vi "Rabi.vi"() -> ()   [LabVIEW 2017]
uses:
  Expose/Labview/Parameters/ExposeParameterBindingType.ctl
  Experiment/ExpGet.vi
  Expose/Labview/Core/ExposeInvokeMethod.vi
  <userlib>/_OpenG.lib/lvdata/lvdata.llb/Get Default Data from Variant__ogtk.vi
panel:
  in  "btnAbort":bool
  in  "btnRunRabi":bool
  in  "Results":T1
  in  "ScanProperties":T2={"PiStartT"=0.0, "PiEndT"=1.0, "N"=100.0, "RepCount"=100, "DoAvg"=TRUE} caption="Scan" {"RepCount" min=1 max=10000000; "N" min=0.0 step=0.1; "PiEndT" min=0.0 step=0.1; "PiStartT" min=0.0 step=0.1}
  in  "RFProperties":cluster{"Amplitude":dbl, "Frequency":dbl}={"Amplitude"=-30.0, "Frequency"=0.0} caption="RF" {"Frequency" min=0.0; "Amplitude" max=12.0}
  in  "SystemConfig":T3={"MTriggerChannel"=1, "FGTriggerChannel"=2, "UseFG"=TRUE, "UseLaser"=TRUE, "UseRF"=TRUE, "LaserChannel"=3, "RFChannel"=4, "UseAnalogInputA0"=FALSE} caption="System" {"RFChannel" min=1 max=32 step=1; "LaserChannel" min=1 max=32 step=1; "FGTriggerChannel" min=1 max=32 step=1; "MTriggerChannel" min=1 max=32 step=1}
  in  "GateDisplay":cluster{"amp":dbl[][], "dt":dbl}
  in  "ReaderProperties":cluster{"BinsPerFreq":u32, "MaxFreq":dbl}={"BinsPerFreq"=1, "MaxFreq"=100000000.0} caption="Reader" {"MaxFreq" min=0.0 step=0.1; "BinsPerFreq" min=1 max=10000}
  in  "TimeProperties":T4={"InitT"=3.0, "WaitForPI"=0.5, "ReadT"=0.25, "WaitAfterPI"=0.5, "WaitForReferenceT"=2.0, "ReadLaserT"=5.0, "WaitAfterMeasurement"=2.0, "LaserDelay"=5.0} caption="Rabi Times" {"LaserDelay" min=0.0 step=0.1; "WaitAfterMeasurement" min=0.0 step=0.1; "ReadLaserT" min=0.0 step=0.1; "WaitForReferenceT" min=0.0 step=0.1; "WaitAfterPI" min=0.0 step=0.1; "ReadT" min=0.0 step=0.1; "WaitForPI" min=0.0 step=0.1; "InitT" min=0.0 step=0.1}
  out "LastBinIndex":dbl caption="#" format="%_7g"
  out "PendingRepetitionCount":dbl caption="Rem." format="%_7g"
  out "BinIndexIndicator":dbl(slide) max=201.0 step=1.0 scale=0.0..1.0
  out "PendingRepIndcator":dbl(slide) max=3.0 step=1.0 scale=0.0..1.0
  out "GraphYPosition":dbl caption="Y" format="%_7g"
  out "GraphXPosition":dbl caption="X" format="%_7g"
  out "IsWorking":bool=TRUE
  out "ExpID":string="Exp967f258c607eed45caf40f4c3101458dC" caption="Exp. ID (Debug)"
  out "ResultsGraph":T5(graph)
  out "MeanStreamVal":dbl caption="M. Ampl." format="%_7g"
  in  "ReadTickTime":dbl
  out "Stream":dbl[](graph) caption="Counts"
  out "TriggersGraph":digitalwaveform(graph)
  # "[¶ scan goes here]"
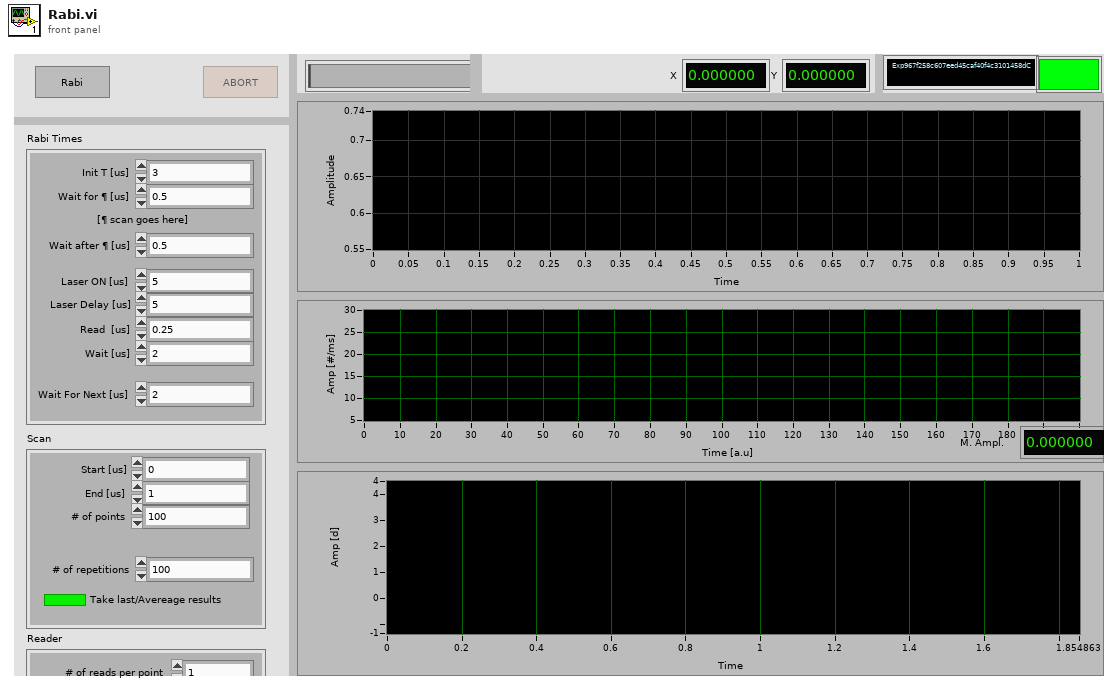
[diagram p1: front panel]
types:
  T1 = cluster{"StepSize":dbl, "Amps":dbl[], "StartOffset":dbl, "Reference":dbl[]}
  T2 = cluster{"PiStartT":dbl, "PiEndT":dbl, "N":dbl, "RepCount":u32, "DoAvg":bool}
  T3 = cluster{"MTriggerChannel":u32, "FGTriggerChannel":u32, "UseFG":bool, "UseLaser":bool, "UseRF":bool, "LaserChannel":u32, "RFChannel":u32, "UseAnalogInputA0":bool}
  T4 = cluster{"InitT":dbl, "WaitForPI":dbl, "ReadT":dbl, "WaitAfterPI":dbl, "WaitForReferenceT":dbl, "ReadLaserT":dbl, "WaitAfterMeasurement":dbl, "LaserDelay":dbl}
  T5 = cluster{dbl, "Frequencies":dbl, "Frequencies":dbl}[]
  T6 = enum8{"Enabled", "Disabled", "Disabled and Grayed Out"}
  T7 = typedef "ExposeParameterBindingType.ctl" = enum16{"ToRemote", "FromRemote", "Bidrectional"}
  T8 = cluster{dbl, "Frequencies":dbl, "Frequencies":dbl}
  T9 = typedef "LVPoint32TypeDef.ctl" = cluster{"Horizontal":i32, "Vertical":i32}
  T10 = typedef "LVRectTypeDef.ctl" = cluster{"Left":i16, "Top":i16, "Right":i16, "Bottom":i16}
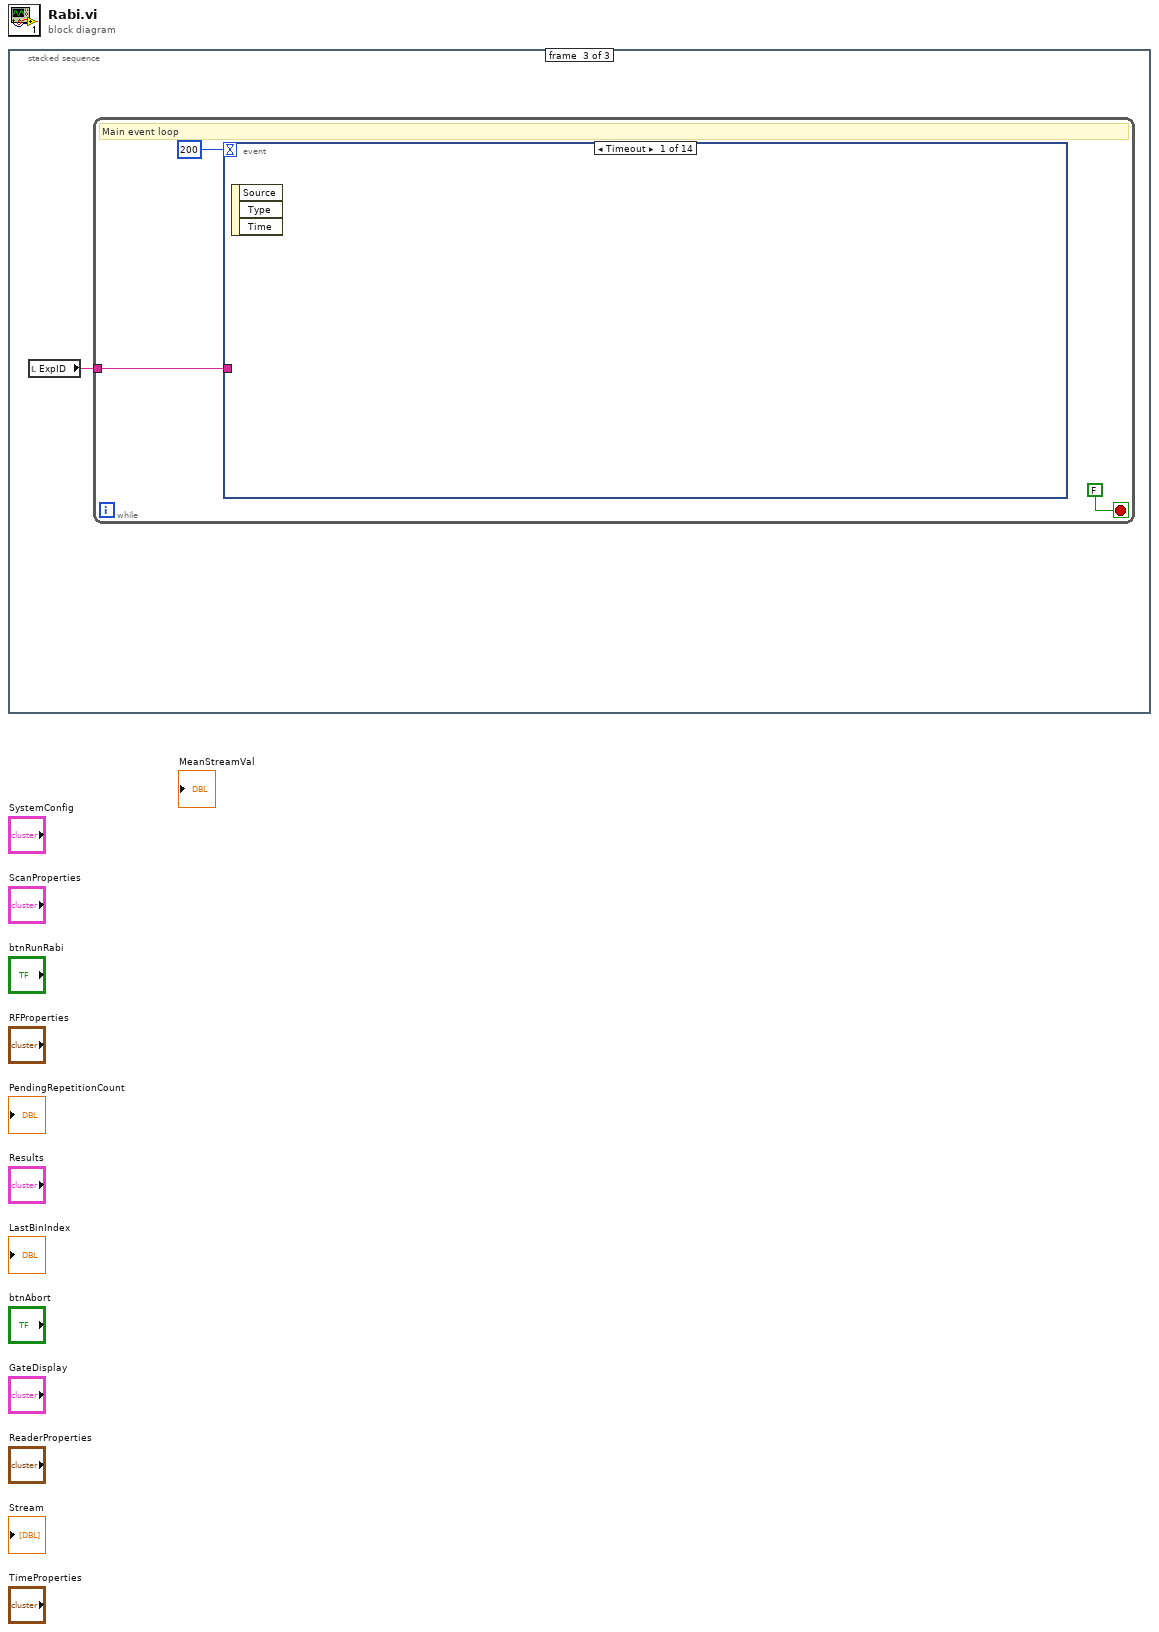
[diagram p0: block diagram]
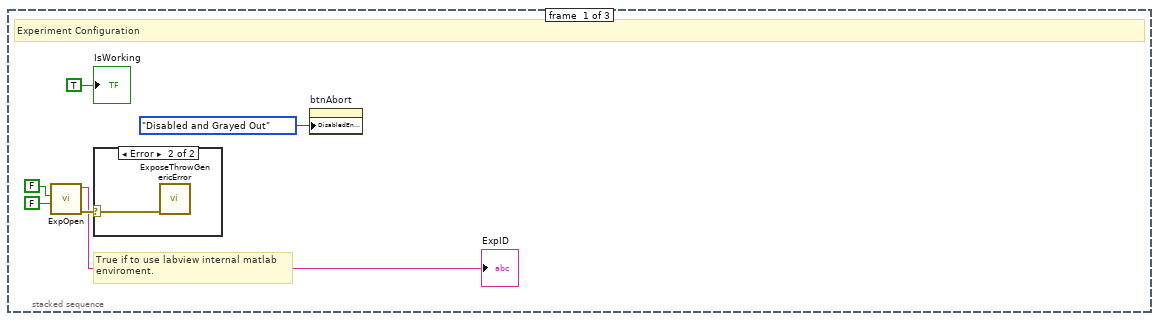
[diagram p2: hidden frame]
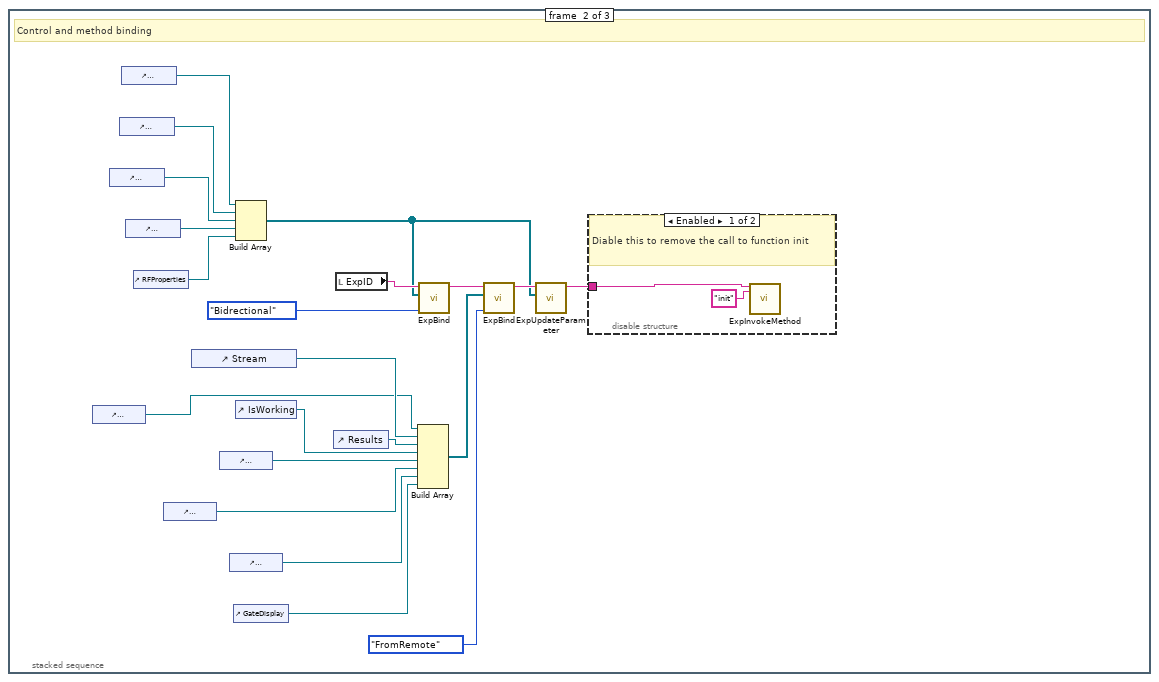
[diagram p4: hidden frame]
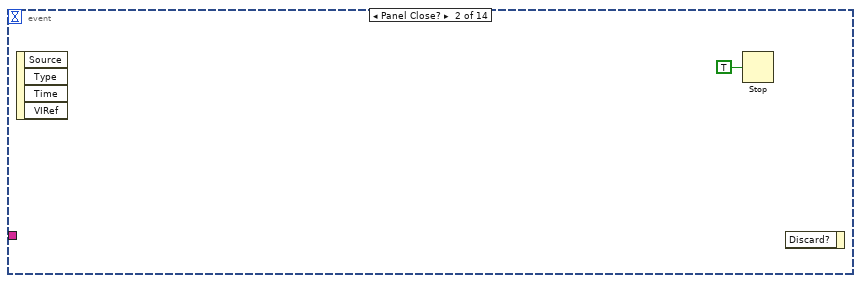
[diagram p6: hidden frame]
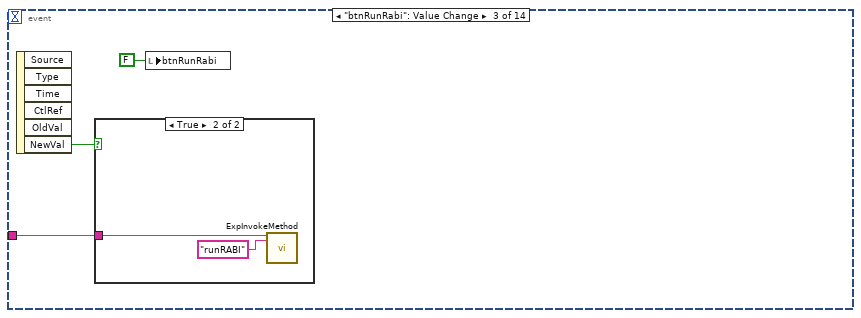
[diagram p7: hidden frame]
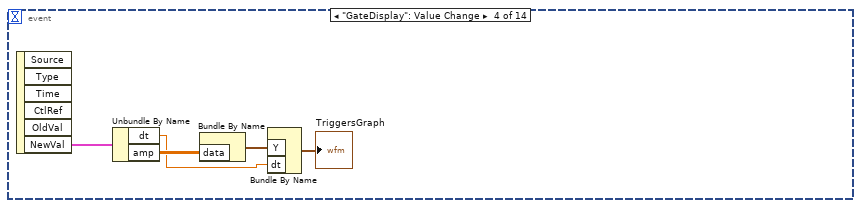
[diagram p9: hidden frame]
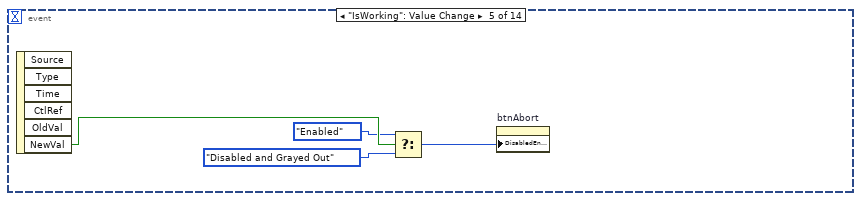
[diagram p10: hidden frame]
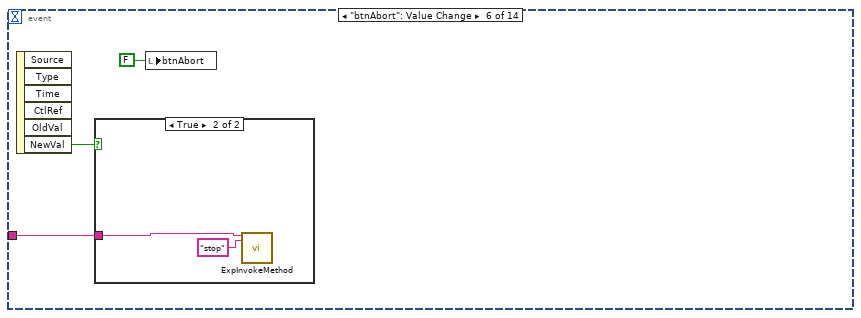
[diagram p11: hidden frame]
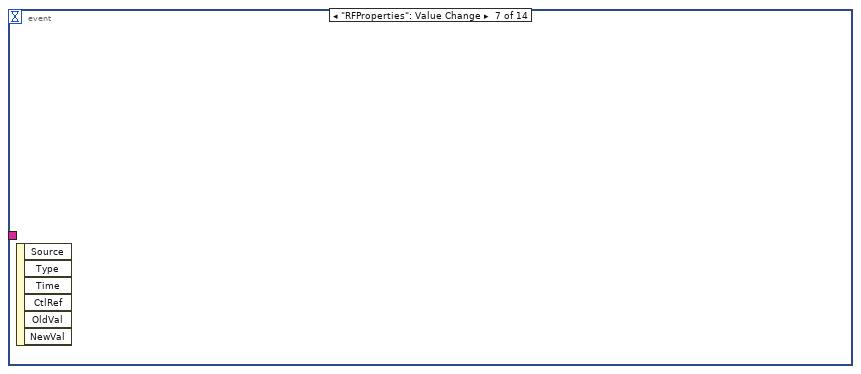
[diagram p13: hidden frame]
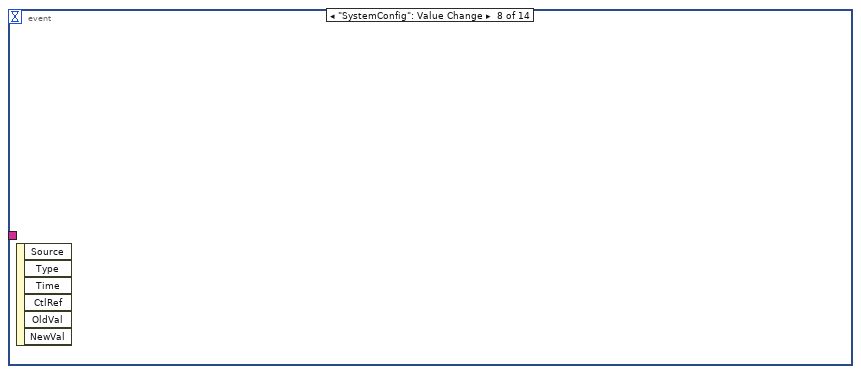
[diagram p14: hidden frame]
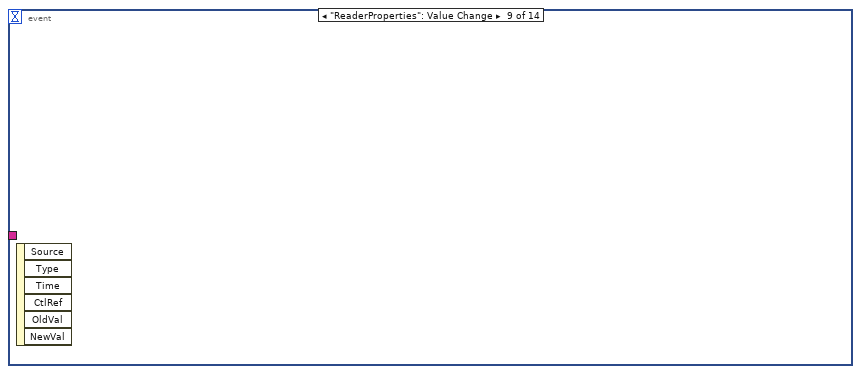
[diagram p15: hidden frame]
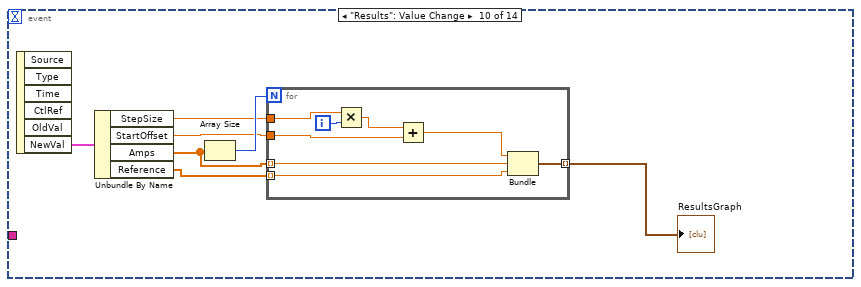
[diagram p16: hidden frame]
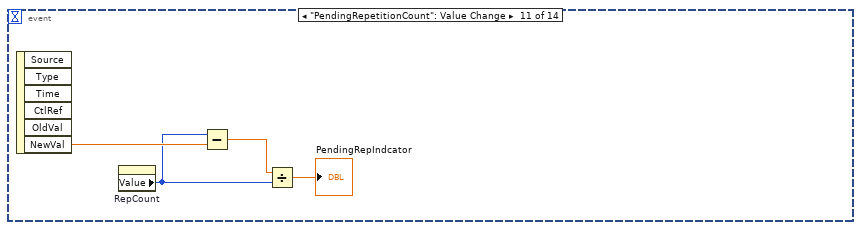
[diagram p17: hidden frame]
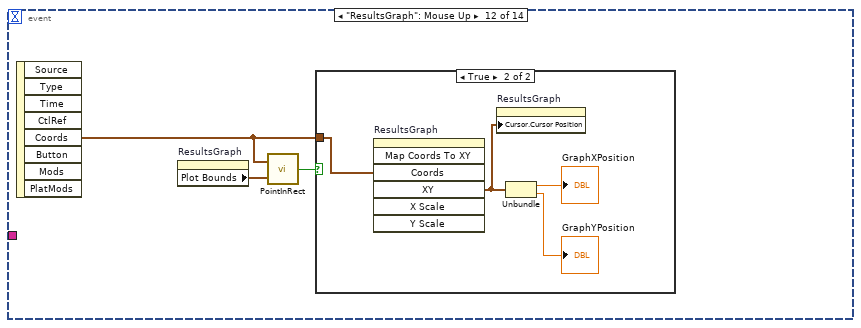
[diagram p18: hidden frame]
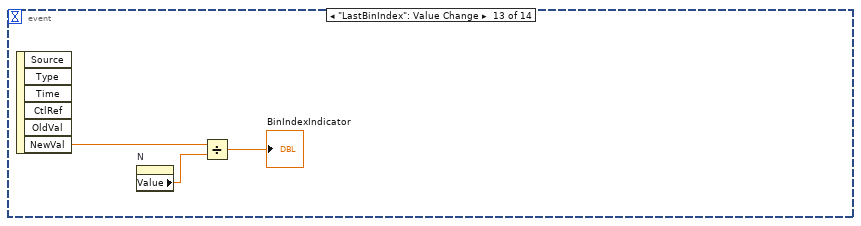
[diagram p20: hidden frame]
diagram:
  n1 = stacked-sequence {
    frame #0 {
      # "True if to use labview internal matlab\nenviroment."
      # "Experiment Configuration"
      n2 = call "ExpOpen.vi"("Do Expose Logging"=FALSE, "Requires Matlab Enviroment"=FALSE) -> ("error out"=w4:errorcluster, "ExpID"=→"ExpID":string)  [unwired: 7 in, 1 out]
      n3 = case shown="Error" w4 {
        selector: w4 -> [_ w7]
        frame No Error {
        }
        frame Error {
          n4 = call "ExposeThrowGenericError.vi"("error in (no error)"=w7) -> ()  [unwired: 10 in, 1 out]
        }
      }
      n5 = property on="btnAbort" class="Bool (strict)"("DisabledEnum"=T6."Disabled and Grayed Out" ("Disabled")) -> ()  [unwired: 2 in, 2 out]
      "IsWorking" <- TRUE ("IsWorking")
    }
    frame #1 {
      # "Control and method binding"
      n6 = control-ref of="MeanStreamVal"() -> (w8:refnum<vi>)
      n7 = control-ref of="ReaderProperties"() -> (w19:refnum<vi>)
      n8 = control-ref of="TimeProperties"() -> (w18:refnum<vi>)
      n9 = control-ref of="ScanProperties"() -> (w10:refnum<vi>)
      n10 = control-ref of="SystemConfig"() -> (w12:refnum<vi>)
      n11 = control-ref of="RFProperties"() -> (w11:refnum<vi>)
      n12 = control-ref of="PendingRepetitionCount"() -> (w15:refnum<vi>)
      n13 = control-ref of="Stream"() -> (w25:refnum<vi>)
      n14 = control-ref of="ReadTickTime"() -> (w17:refnum<vi>)
      n15 = control-ref of="LastBinIndex"() -> (w14:refnum<vi>)
      n16 = control-ref of="GateDisplay"() -> (w13:refnum<vi>)
      n17 = Build Array(w10, w18, w19, w12, w11) -> (w16:refnum<vi>[])
      n18 = control-ref of="IsWorking"() -> (w23:refnum<vi>)
      n19 = control-ref of="Results"() -> (w9:refnum<vi>)
      n20 = local read "ExpID"() -> (w28:string)
      n21 = Build Array(w8, w25, w9, w23, w17, w15, w14, w13) -> (w24:refnum<vi>[])
      n22 = call "ExpBind.vi"("Binding Type"=ExposeParameterBindingType."Bidrectional", "Value"=w16, "ExpID"=w28) -> ("ExpID out"=w21:string)  [unwired: 7 in, 1 out]
      n23 = call "ExpBind.vi"("Binding Type"=ExposeParameterBindingType."FromRemote", "Value"=w24, "ExpID"=w21) -> ("ExpID out"=w20:string)  [unwired: 7 in, 1 out]
      n24 = call "ExpUpdateParameter.vi"("Variant"=w16, "ExpID"=w20) -> ("ExpID out"=w22:string)  [unwired: 8 in, 1 out]
      n25 = disable-structure shown="Enabled" {
        disable-tunnel: w22 -> [w30 _]
        frame Enabled {
          # "Diable this to remove the call to function init"
          n26 = call "ExpInvokeMethod.vi"("ExpID"=w30, "Method Name"="init") -> ()  [unwired: 15 in, 3 out]
        }
        frame Disabled {
        }
      }
    }
    frame #2 {
      n27 = local read "ExpID"() -> (w31:string)
      n28 = while {
        tunnel: w31 -> [w32]
        stop <- FALSE stop-if-true
        # "Main event loop"
        n29 = event shown="[0] Timeout" {
          selector: _ -> [_ _ _ _ _ _ _ _ _ _ _ _ _ _]
          dyn-events: _ -> [_ _ _ _ _ _ _ _ _ _ _ _ _ _]
          timeout: 200 -> [_ _ _ _ _ _ _ _ _ _ _ _ _ _]
          tunnel: w32 -> [_ _ w38 _ _ w51 _ _ _ _ _ _ _ _]
          event Timeout {
            n30 = event-data() -> ()  [unwired: 1 in, 3 out]
          }
          event Panel Close? {
            n31 = event-data() -> ()  [unwired: 1 in, 4 out]
            n32 = Stop(stop? (T)=TRUE) -> ()
            n33 = event-data() -> ()  [unwired: 2 in, 1 out]
          }
          event "btnRunRabi": Value Change {
            n34 = event-data() -> ("NewVal"=w37:bool)  [unwired: 1 in, 5 out]
            n35 = case shown="True" w37 {
              tunnel: w38 -> [_ w40]
              frame False {
              }
              frame True {
                n36 = call "ExpInvokeMethod.vi"("ExpID"=w40, "Method Name"="runRABI") -> ()  [unwired: 15 in, 3 out]
              }
            }
            n37 = local write "btnRunRabi"(FALSE ("btnRunOdmr")) -> ()
          }
          event "GateDisplay": Value Change {
            n38 = event-data() -> ("NewVal"=w45:cluster{"amp":dbl[][], "dt":dbl})  [unwired: 1 in, 5 out]
            n39 = Unbundle By Name(w45) -> ("dt"=w43:dbl, "amp"=w44:dbl[][])
            n40 = Bundle By Name("data"=w44) -> (w42:digitaldata)  [unwired: 1 in]
            n41 = Bundle By Name("Y"=w42, "dt"=w43) -> (→"TriggersGraph":digitalwaveform)  [unwired: 1 in]
          }
          event "IsWorking": Value Change {
            n42 = event-data() -> ("NewVal"=w49:bool)  [unwired: 1 in, 5 out]
            n43 = Select(t=T6."Enabled" ("Disabled"), s=w49, f=T6."Disabled and Grayed Out" ("Disabled")) -> (s? t:f=w46:T6)
            n44 = property on="btnAbort" class="Bool (strict)"("DisabledEnum"=w46) -> ()  [unwired: 2 in, 2 out]
          }
          event "btnAbort": Value Change {
            n45 = event-data() -> ("NewVal"=w52:bool)  [unwired: 1 in, 5 out]
            n46 = case shown="True" w52 {
              tunnel: w51 -> [_ w54]
              frame False {
              }
              frame True {
                n47 = call "ExpInvokeMethod.vi"("ExpID"=w54, "Method Name"="stop") -> ()  [unwired: 15 in, 3 out]
              }
            }
            n48 = local write "btnAbort"(FALSE ("btnAbort")) -> ()
          }
          event "RFProperties": Value Change {
            n49 = event-data() -> ()  [unwired: 1 in, 6 out]
          }
          event "SystemConfig": Value Change {
            n50 = event-data() -> ()  [unwired: 1 in, 6 out]
          }
          event "ReaderProperties": Value Change {
            n51 = event-data() -> ()  [unwired: 1 in, 6 out]
          }
          event "Results": Value Change {
            n52 = event-data() -> ("NewVal"=w61:T1)  [unwired: 1 in, 5 out]
            n53 = Unbundle By Name(w61) -> ("StepSize"=w58:dbl, "StartOffset"=w59:dbl, "Amps"=w57:dbl[], "Reference"=w56:dbl[])
            n54 = Array Size(array=w57) -> (size(s)=w60:i32)
            n55 = for {
              N: w60 -> [_]
              tunnel: w59 -> [w69]
              tunnel: w58 -> [w67]
              tunnel: w57 -> [w65] mode=indexing
              tunnel: w56 -> [w62] mode=indexing
              tunnel: [w64] -> w55 mode=indexing
              i -> [w68]
              n56 = Multiply(x=w67, y=w68) -> (x*y=w66:dbl)
              n57 = Add(x=w66, y=w69) -> (x+y=w63:dbl)
              n58 = Bundle(w63, "Frequencies"=w65, "Frequencies"=w62) -> (w64:T8)  [unwired: 1 in]
            }
            "ResultsGraph" <- w55
          }
          event "PendingRepetitionCount": Value Change {
            n59 = event-data() -> ("NewVal"=w73:dbl)  [unwired: 1 in, 5 out]
            n60 = property on="RepCount" class="DigNum (strict)"() -> ("Value"=w71:u32)  [unwired: 2 in, 2 out]
            n61 = Subtract(x=w71, y=w73) -> (x-y=w72:dbl)
            n62 = Divide(x=w72, y=w71) -> (x/y=→"PendingRepIndcator":dbl)
          }
          event "ResultsGraph": Mouse Up {
            n63 = event-data() -> ("Coords"=w75:T9)  [unwired: 1 in, 7 out]
            n64 = property on="ResultsGraph" class="XYGraph (strict)"() -> ("Plot Bounds"=w76:T10)  [unwired: 2 in, 2 out]
            n65 = call <vilib>:"PointInRect.vi"("rect"=w76, "point"=w75) -> ("pt in rect"=w74:bool)
            n66 = case shown="True" w74 {
              tunnel: w75 -> [_ w80]
              frame False {
              }
              frame True {
                n67 = invoke on="ResultsGraph" class="XYGraph (strict)" method="Map Coords To XY"("Coords"=w80) -> ("XY"=w79:cluster{"X":dbl, "Y":dbl})  [unwired: 6 in, 6 out]
                n68 = property on="ResultsGraph" class="XYGraph (strict)"("Cursor.Cursor Position"=w79) -> ()  [unwired: 2 in, 2 out]
                n69 = Unbundle(w79) -> ("X"=→"GraphXPosition":dbl, "Y"=→"GraphYPosition":dbl)
              }
            }
          }
          event "LastBinIndex": Value Change {
            n70 = event-data() -> ("NewVal"=w83:dbl)  [unwired: 1 in, 5 out]
            n71 = property on="N" class="DigNum (strict)"() -> ("Value"=w81:dbl)  [unwired: 2 in, 2 out]
            n72 = Divide(x=w83, y=w81) -> (x/y=→"BinIndexIndicator":dbl)
          }
          event "ReadTickTime": Value Change {
            n73 = event-data() -> ()  [unwired: 1 in, 6 out]
            n74 = property on="Stream" class="WFGraph (strict)"("XScale.Multiplier"="ReadTickTime") -> ()  [unwired: 2 in, 2 out]
          }
        }
      }
    }
  }
